vi "Write Delay Method.vi"(10 "Delay Method":T1, 11 "Abstract Delay Line in":refnum<class "Abstract Delay Line.lvclass">) -> (3 "Abstract Delay Line out":refnum<class "Abstract Delay Line.lvclass">)   [LabVIEW 2016, in "_Delay Line.lvlib" / "Abstract Delay Line.lvclass"]
uses:
  Abstract Delay Line.lvclass
  Typedef/Delay Method.ctl
  Abstract Delay Line.lvclass/Abstract Delay Line.ctl
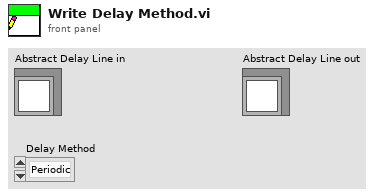
[diagram p1: front panel]
types:
  T1 = typedef "_Delay Line.lvlib/Abstract Delay Line.lvclass/Delay Method.ctl" = enum8{"Periodic", "Fixed"}
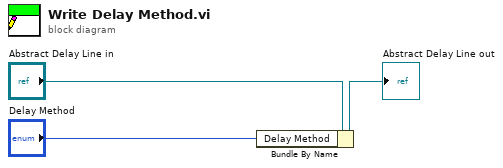
[diagram p0: block diagram]
diagram:
  n1 = Bundle By Name(cluster="Abstract Delay Line in", "Delay Method"="Delay Method") -> (→"Abstract Delay Line out":refnum<class "Abstract Delay Line.lvclass">)
